vi "Initialize Frame.vi"(8 "Error In":errorcluster, 10 "Size":T1, 11 "Display In":refnum<class "Display.lvclass">) -> (0 "Error Out":errorcluster, 3 "Display Out":refnum<class "Display.lvclass">)   [LabVIEW 2019, in "Display.lvclass"]
uses:
  Display.lvclass
  Controls/Size.ctl
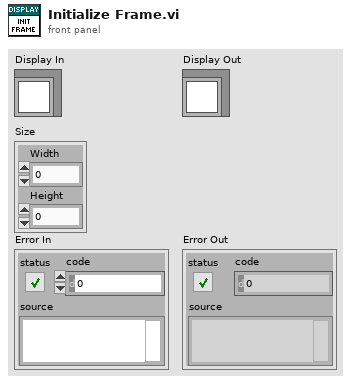
[diagram p1: front panel]
types:
  T1 = typedef "Display.lvclass/Size.ctl" = cluster{"Width":i32, "Height":i32}
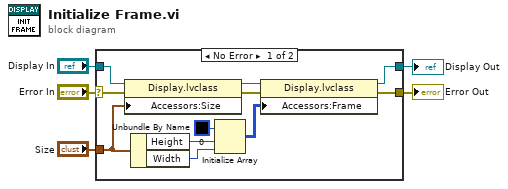
[diagram p0: block diagram]
diagram:
  n1 = case shown="No Error" "Error In" {
    selector: "Error In" -> [w16 w17]
    tunnel: "Display In" -> [w15 w18]
    tunnel: [w6 w18] -> w3
    tunnel: [w14 w17] -> w2
    tunnel: "Size" -> [w12 _]
    frame No Error {
      n2 = property class="Display.lvclass"(reference=w15, error in=w16, "Accessors:Size"=w12) -> (reference out=w7:refnum<class "Display.lvclass">, error out=w8:errorcluster)
      n3 = Unbundle By Name(w12) -> ("Height"=w11:i32, "Width"=w10:i32)
      n4 = Initialize Array(u32 0 ("Color"), w11, w10) -> (w9:u32[][])
      n5 = property class="Display.lvclass"(reference=w7, error in=w8, "Accessors:Frame"=w9) -> (reference out=w6:refnum<class "Display.lvclass">, error out=w14:errorcluster)
    }
    frame Error {
    }
  }
  "Display Out" <- w3
  "Error Out" <- w2
